vi "Flat Sequence.vi"() -> ()   [LabVIEW 2024]
panel:
  in  "Timer 3":u32
  out "LED 3":bool
  in  "Control 3":bool
  in  "Timer 2":u32
  out "LED 2":bool
  in  "Control 2":bool
  in  "Timer 1":u32
  out "LED 1":bool
  in  "Control 1":bool
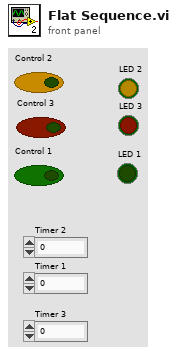
[diagram p1: front panel]
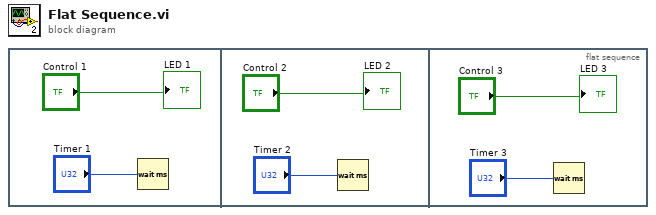
[diagram p0: block diagram]
diagram:
  n1 = flat-sequence {
    frame #0 {
      n2 = Wait (ms)(milliseconds to wait="Timer 1") -> ()  [unwired: 1 out]
      "LED 1" <- "Control 1"
    }
    frame #1 {
      n3 = Wait (ms)(milliseconds to wait="Timer 2") -> ()  [unwired: 1 out]
      "LED 2" <- "Control 2"
    }
    frame #2 {
      n4 = Wait (ms)(milliseconds to wait="Timer 3") -> ()  [unwired: 1 out]
      "LED 3" <- "Control 3"
    }
  }
